vi "Equal.vi"(8 "error in (no error)":errorcluster caption="错误输入（无错误）", 10 "Dictionary":refnum<class "Dictionary.lvclass"> caption="DNL_LabVIEW Object in", 11 "Dictionary In":refnum<class "Dictionary.lvclass"> caption="DNL_LabVIEW Object in") -> (0 "error out":errorcluster caption="错误输出", 1 "Equal":bool, 3 "Dictionary Out":refnum<class "Dictionary.lvclass"> caption="DNL_LabVIEW Object out")   [LabVIEW 2012, in "Dictionary.lvclass"]
uses:
  Dictionary.lvclass
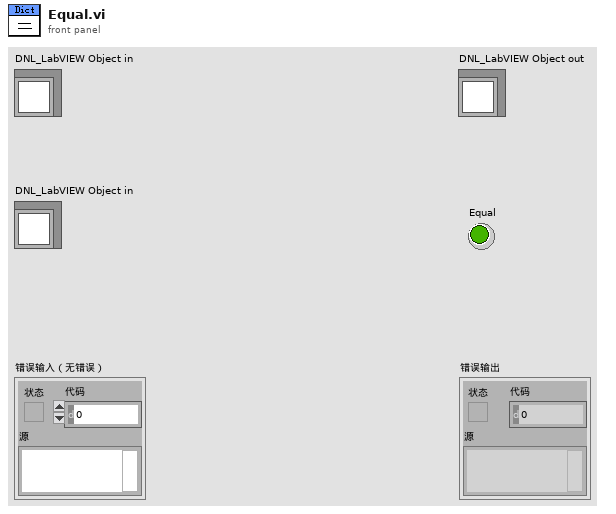
[diagram p1: front panel]
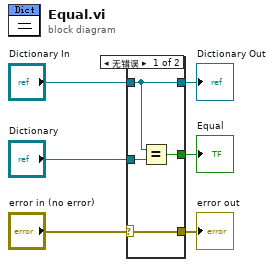
[diagram p0: block diagram]
diagram:
  n1 = case shown="无错误" "error in (no error)" {
    selector: "error in (no error)" -> [w10 w12]
    tunnel: [w10 w12] -> w5
    tunnel: [w8 w11] -> w3
    tunnel: "Dictionary In" -> [w8 w11]
    tunnel: "Dictionary" -> [w9 _]
    tunnel: [w7 _] -> w1
    frame No Error {
      n2 = Equal?(x=w8, y=w9) -> (x = y?=w7:bool)
    }
    frame Error {
    }
  }
  "error out" <- w5
  "Dictionary Out" <- w3
  "Equal" <- w1
